vi "Get CMY Components.vi"(0 "CMY Color in":refnum<class "CMY Color.lvclass">, 11 "error in (no error)":errorcluster) -> (4 "CMY Color out":refnum<class "CMY Color.lvclass">, 6 "C":u8, 8 "M":u8, 10 "Y":u8, 15 "error out":errorcluster)   [LabVIEW 2020, in "CMY Color.lvclass"]
doc: "Get the cyan, magenta and yellow components of a CMY color"
uses:
  CMY Color.lvclass
  CMY Color.lvclass/CMY Color.ctl
panel:
  # "expressionflow.com"
  # "Copyright (c) 2008 Tomi Maila. All rights reserved."
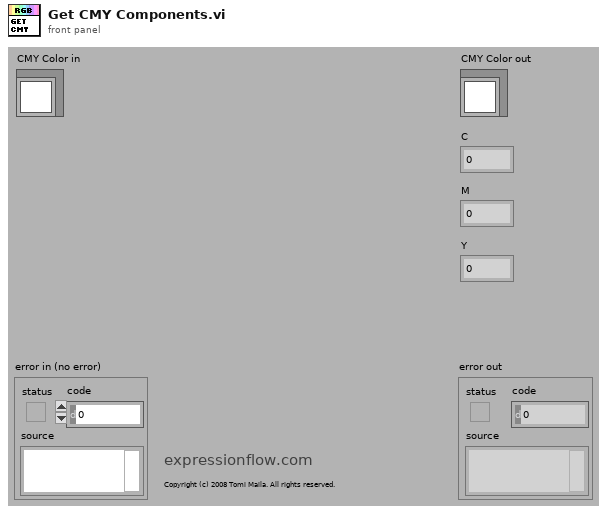
[diagram p1: front panel]
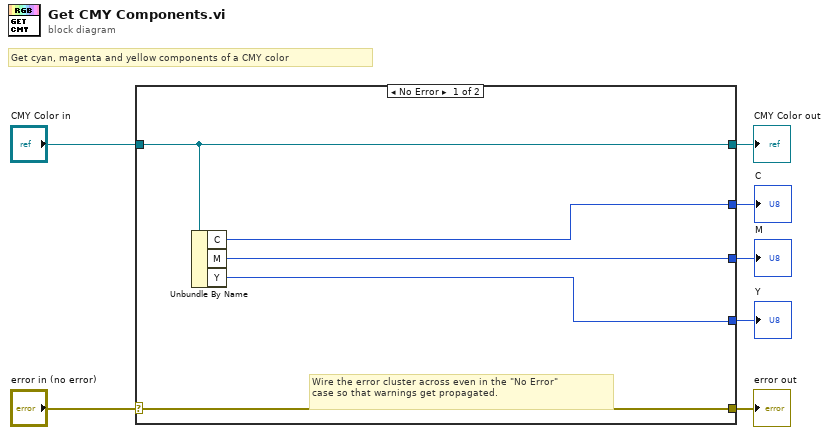
[diagram p0: block diagram]
diagram:
  # "Get cyan, magenta and yellow components of a CMY color"
  n1 = case shown="No Error" "error in (no error)" {
    selector: "error in (no error)" -> [w12 w14]
    tunnel: [w12 w14] -> w6
    tunnel: [w11 w13] -> w4
    tunnel: "CMY Color in" -> [w11 w13]
    tunnel: [w10 _] -> w3
    tunnel: [w9 _] -> w2
    tunnel: [w8 _] -> w1
    frame No Error {
      # "Wire the error cluster across even in the \"No Error\"\ncase so that warnings get propagated."
      n2 = Unbundle By Name(w11) -> ("C"=w10:u8, "M"=w9:u8, "Y"=w8:u8)
    }
    frame Error {
    }
  }
  "error out" <- w6
  "CMY Color out" <- w4
  "C" <- w3
  "M" <- w2
  "Y" <- w1
